vi "Search String Array Output Index.vi"(10 "Search Expression":string, 11 "filenames":string[](array[string])) -> (3 "Array":i32[](array[numeric]))   [LabVIEW 2012]
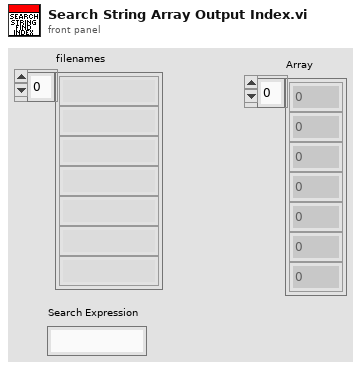
[diagram p1: front panel]
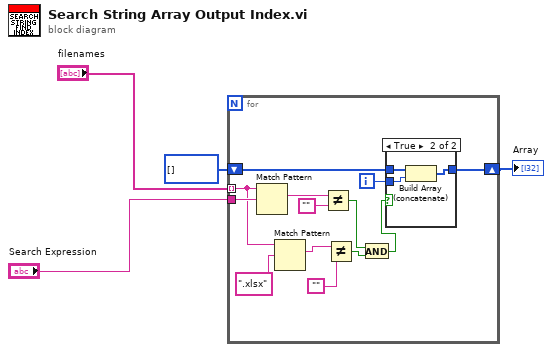
[diagram p0: block diagram]
diagram:
  n1 = for {
    tunnel: "filenames" -> [w11] mode=indexing
    shift-right: [w13] -> w3
    shift-left: i32[] [] -> [w15]
    tunnel: "Search Expression" -> [w12]
    i -> [w14]
    n2 = Match Pattern(string=w11, regular expression=w12) -> (match substring=w16:string)  [unwired: 1 in, 3 out]
    n3 = Match Pattern(string=w11, regular expression=".xlsx") -> (match substring=w9:string)  [unwired: 1 in, 3 out]
    n4 = Not Equal?(x=w16, y="") -> (x != y?=w7:bool)
    n5 = Not Equal?(x=w9, y="") -> (x != y?=w6:bool)
    n6 = And(x=w7, y=w6) -> (x .and. y?=w5:bool)
    n7 = case shown="True" w5 {
      tunnel: w15 -> [w18 w21]
      tunnel: w14 -> [_ w20]
      tunnel: [w18 w19] -> w13
      frame False {
      }
      frame True {
        n8 = Build Array (concatenate)(w21, w20) -> (w19:i32[])
      }
    }
  }
  "Array" <- w3
